vi "Multimeter handler.vi"(8 "error in (no error)":errorcluster, 11 "Message Queues out":T1) -> (0 "error out":errorcluster, 3 "Message Queue":refnum<queue>)   [LabVIEW 2014]
uses:
  support/Message Queue/Message Queue.lvlib
  support/Message Queue/Enqueue Message (Single).vi
  Engine/Message.ctl
  Teszt/Teszt.ctl
  Teszt/Command.ctl
  <vilib>/ErrorRing/Error Ring.xnode
  <vilib>/Utility/error.llb/Error Cluster From Error Code.vi
  support/Message Queue/Message Cluster.ctl
  support/Message Queue/All Message Queues.ctl
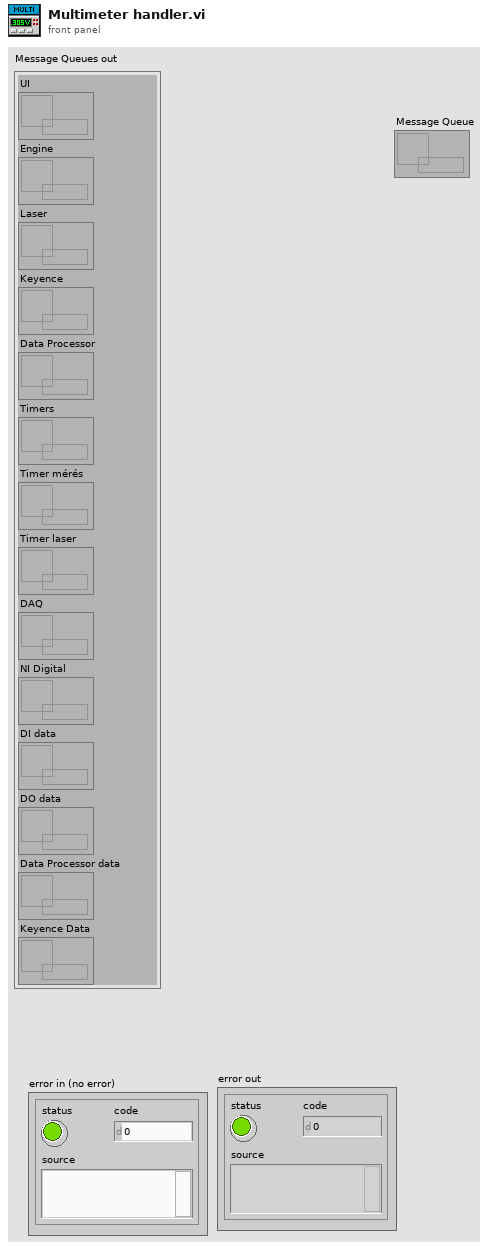
[diagram p1: front panel]
types:
  T1 = typedef "Message Queue.lvlib/All Message Queues.ctl" = cluster{"UI":refnum<queue>, "Engine":refnum<queue>, "Laser":refnum<queue>, "Keyence":refnum<queue>, "Data Processor":refnum<queue>, "Timers":refnum<queue>, "Timer mérés":refnum<queue>, "Timer laser":refnum<queue>, "DAQ":refnum<queue>, "NI Digital":refnum<queue>, "DI data":refnum<queue>, "DO data":refnum<queue>, "Data Processor data":refnum<queue>, "Keyence Data":refnum<queue>}
  T2 = typedef "Teszt.ctl" = cluster{"Thread ID":dbl, "Mérésszám":string, "Mérés/Utasítás":string, "Command":T3, "Min":string, "Max":string, "Aktív?":bool, "Log?":bool, "Kiértékelés":bool, "Etalon 1 exp":bool, "Etalon 2 exp":bool, "Etalon 3 exp":bool, "Etalon 4 exp":bool, "Etalon 5 exp":bool}
  T3 = typedef "Command.ctl" = cluster{"Parancs":string, "Paraméter 1":string, "Paraméter 2":string, "Paraméter 3":string, "Paraméter 4":string, "Paraméter 5":string, "Eredmény":string}
  T4 = typedef "Message.ctl" = cluster{"Thread ID":u16, "Callback":string, "Data":variant, "Error":errorcluster}
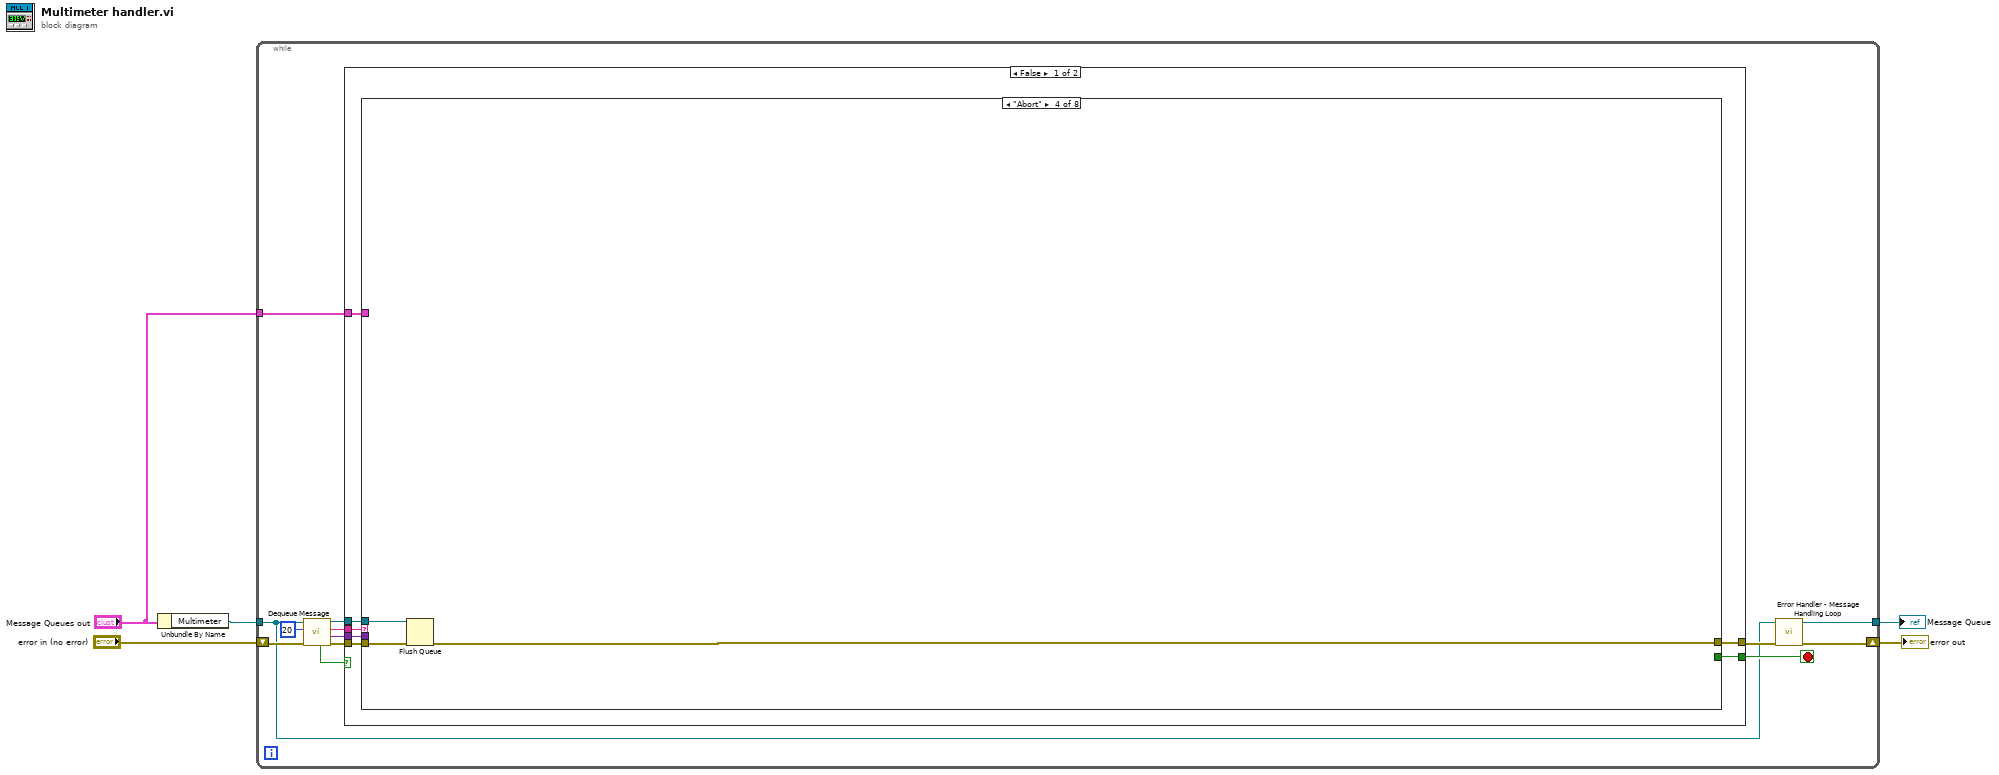
[diagram p0: block diagram]
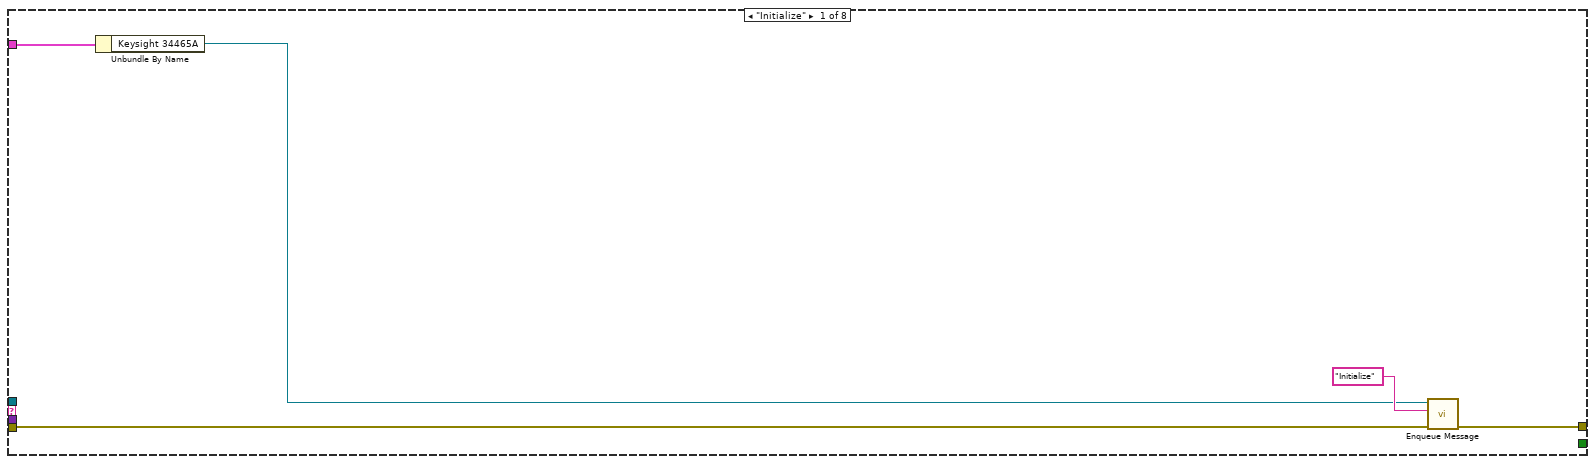
[diagram p2: hidden frame]
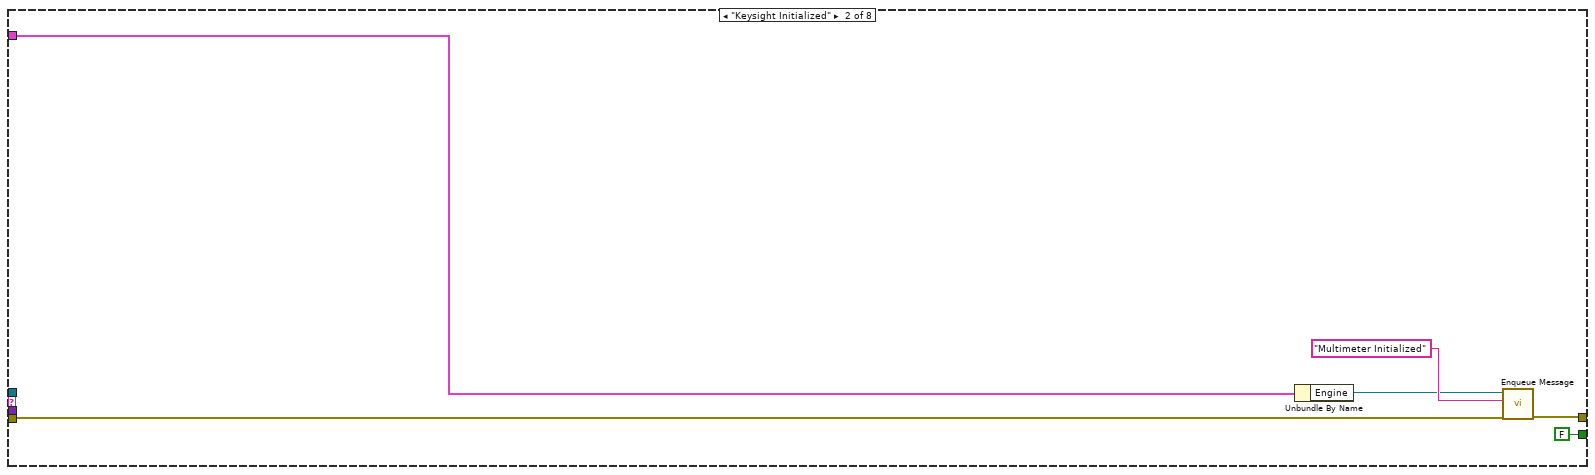
[diagram p3: hidden frame]
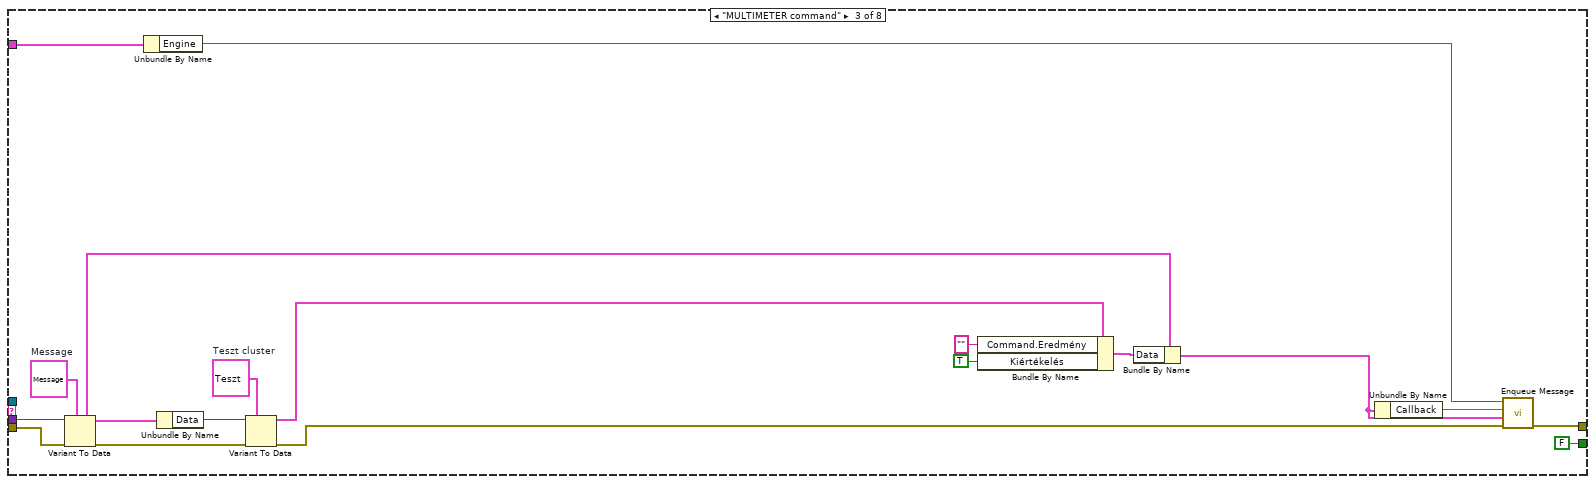
[diagram p4: hidden frame]
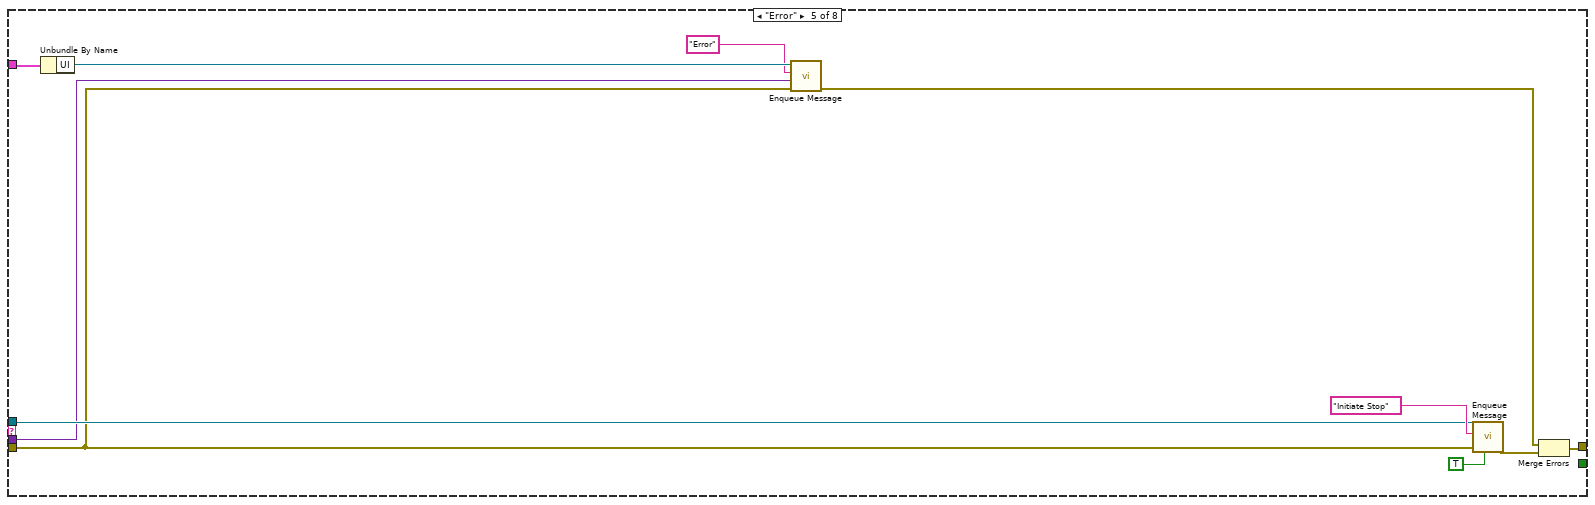
[diagram p5: hidden frame]
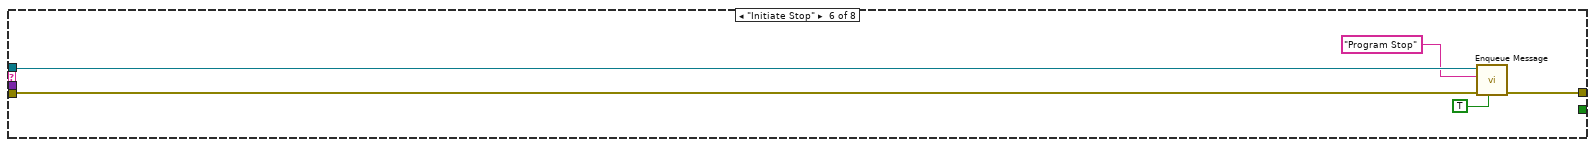
[diagram p6: hidden frame]
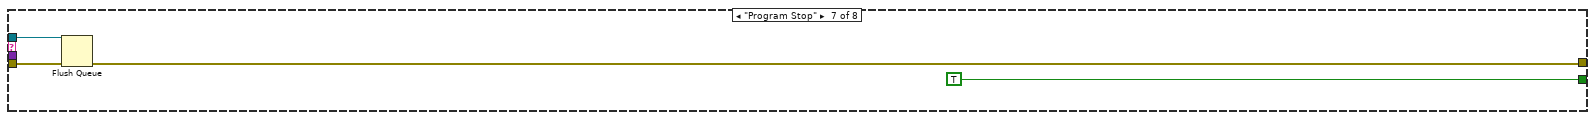
[diagram p7: hidden frame]
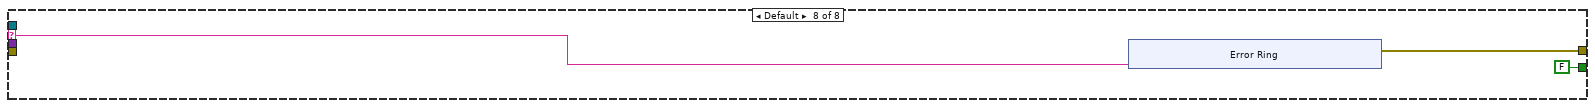
[diagram p8: hidden frame]
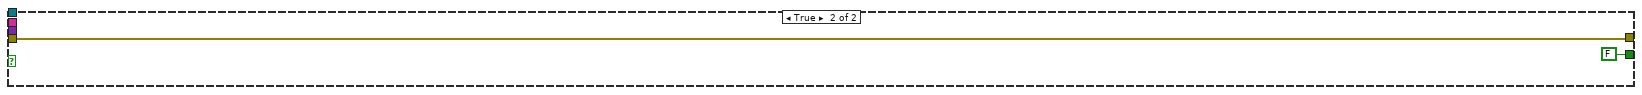
[diagram p9: hidden frame]
diagram:
  n1 = Unbundle By Name("Message Queues out") -> ("Multimeter"=w2:refnum<queue>)
  n2 = while {
    tunnel: w2 -> [w6]
    shift-right: [w10] -> w5
    shift-left: "error in (no error)" -> [w18]
    tunnel: "Message Queues out" -> [w8]
    tunnel: [w7] -> w1
    stop <- w14 stop-if-true
    n3 = call "Dequeue Message.vi"("error in (no error)"=w18, "timeout in ms (-1)"=20, "Message Queue"=w6) -> ("error out"=w16:errorcluster, "Message Data"=w11:variant, "Message"=w17:string, "dup Message Queue"=w15:refnum<queue>, "timed out?"=w12:bool)  [unwired: 4 in]
    n4 = case shown="False" w12 {
      tunnel: w17 -> [w25 _]
      tunnel: w16 -> [w24 w88]
      tunnel: w15 -> [w23 _]
      tunnel: [w22 FALSE] -> w14
      tunnel: [w21 w88] -> w9
      tunnel: w11 -> [w20 _]
      tunnel: w8 -> [w19 _]
      frame False {
        n5 = case shown="\"Abort\"" w25 {
          selector: w25 -> [_ _ _ _ _ _ _ w78]
          tunnel: w24 -> [w28 w31 w46 w57 w58 w72 w75 _]
          tunnel: w23 -> [_ _ _ w56 w61 w71 w77 _]
          tunnel: [w29 w35 w53 w55 w62 w73 w74 w79] -> w21
          tunnel: [_ FALSE FALSE _ _ _ TRUE FALSE] -> w22
          tunnel: w20 -> [_ _ w45 _ w59 _ _ _]
          tunnel: w19 -> [w27 w32 w51 _ w60 _ _ _]
          frame "Initialize" {
            n6 = Unbundle By Name(w27) -> ("Keysight 34465A"=w26:refnum<queue>)
            n7 = call-poly "Enqueue Message.vi"("error in (no error)"=w28, "Message"="Initialize", "Message Queue"=w26) -> ("error out"=w29:errorcluster)  [unwired: 7 in, 1 out]
          }
          frame "Keysight Initialized" {
            n8 = Unbundle By Name(w32) -> ("Engine"=w33:refnum<queue>)
            n9 = call-poly "Enqueue Message.vi"("error in (no error)"=w31, "Message"="Multimeter Initialized", "Message Queue"=w33) -> ("error out"=w35:errorcluster)  [unwired: 7 in, 1 out]
          }
          frame "MULTIMETER command" {
            w47 = T2 {"Thread ID"=0.0, "Mérésszám"="", "Mérés/Utasítás"="", "Command"={"Parancs"="", "Paraméter 1"="", "Paraméter 2"="", "Paraméter 3"="", "Paraméter 4"="", "Paraméter 5"="", "Eredmény"=""}, "Min"="", "Max"="", "Aktív?"=FALSE, "Log?"=FALSE, "Kiértékelés"=FALSE, "Etalon 1 exp"=FALSE, "Etalon 2 exp"=FALSE, "Etalon 3 exp"=FALSE, "Etalon 4 exp"=FALSE, "Etalon 5 exp"=FALSE}  # Teszt cluster
            w50 = T4 {"Thread ID"=0, "Callback"="", "Data"=variant, "Error"={"status"=FALSE, "code"=0, "source"=""}}  # Message
            n10 = Variant To Data(error in=w46, type=w50, Variant=w45) -> (data=w41:T4, error out=w49:errorcluster)
            n11 = Unbundle By Name(w51) -> ("Engine"=w52:refnum<queue>)
            n12 = Unbundle By Name(w41) -> ("Data"=w48:variant)
            n13 = Variant To Data(error in=w49, type=w47, Variant=w48) -> (data=w37:T2, error out=w40:errorcluster)
            n14 = Bundle By Name(cluster=w37, "Command.Eredmény"="", "Kiértékelés"=TRUE) -> (w44:T2)
            n15 = Bundle By Name(cluster=w41, "Data"=w44) -> (w42:T4)
            n16 = Unbundle By Name(w42) -> ("Callback"=w43:string)
            n17 = call-poly "Enqueue Message.vi"("error in (no error)"=w40, "Message Data"=w42, "Message"=w43, "Message Queue"=w52) -> ("error out"=w53:errorcluster)  [unwired: 6 in, 1 out]
          }
          frame "Abort" {
            n18 = Flush Queue(queue=w56, error in (no error)=w57) -> (error out=w55:errorcluster)  [unwired: 2 out]
          }
          frame "Error" {
            n19 = Unbundle By Name(w60) -> ("UI"=w65:refnum<queue>)
            n20 = call-poly "Enqueue Message.vi"("error in (no error)"=w58, "Message Data"=w59, "Message"="Error", "Message Queue"=w65) -> ("error out"=w67:errorcluster)  [unwired: 6 in, 1 out]
            n21 = call-poly "Enqueue Message.vi"("Priority Message? (F)"=TRUE, "error in (no error)"=w58, "Message"="Initiate Stop", "Message Queue"=w61) -> ("error out"=w66:errorcluster)  [unwired: 6 in, 1 out]
            n22 = Merge Errors(w67, w66) -> (w62:errorcluster)
          }
          frame "Initiate Stop" {
            n23 = call-poly "Enqueue Message.vi"("Priority Message? (F)"=TRUE, "error in (no error)"=w72, "Message"="Program Stop", "Message Queue"=w71) -> ("error out"=w73:errorcluster)  [unwired: 6 in, 1 out]
          }
          frame "Program Stop" {
            n24 = Flush Queue(queue=w77, error in (no error)=w75) -> (error out=w74:errorcluster)  [unwired: 2 out]
          }
          frame Default {
            n25 = xnode "Error Ring"("parameter 0"=w78) -> ("error out"=w79:errorcluster)
          }
        }
      }
      frame True {
      }
    }
    n26 = call "Error Handler - Message Handling Loop.vi"("error in (no error)"=w9, "Message Queue"=w6) -> ("dup error in"=w10:errorcluster, "dup Message Queue"=w7:refnum<queue>)  [unwired: 8 in]
  }
  "error out" <- w5
  "Message Queue" <- w1
